vi "SetWavelength.vi"(8 "error in (no error)":errorcluster, 10 "Wavelength, nm":dbl=620.0, 11 "OPA in":refnum<class "OPA.lvclass">) -> (0 "error out":errorcluster, 3 "OPA out":refnum<class "OPA.lvclass">)   [LabVIEW 2017, in "OPA.lvclass"]
uses:
  OPA.lvclass
  Typedefs/PrivateEvents--OPA.SetWavelength.ctl
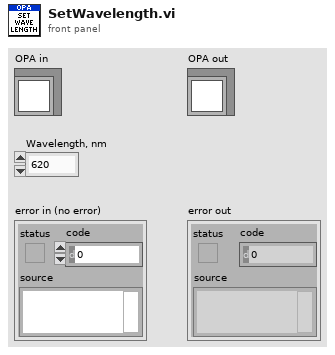
[diagram p1: front panel]
types:
  T1 = typedef "OPA.lvclass/PrivateEvents--OPA.SetWavelength.ctl" = cluster{"Wavelength, nm":dbl}
  T2 = typedef "OPA.lvclass/PrivateEvents--Cluster.ctl" = cluster{"SetWavelength":refnum<user-event>, "SetShutterState":refnum<user-event>}
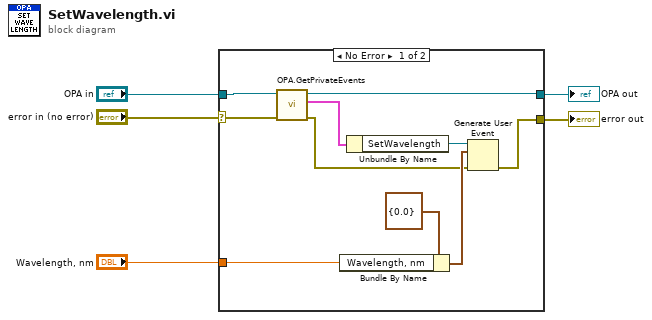
[diagram p0: block diagram]
diagram:
  n1 = case shown="No Error" "error in (no error)" {
    selector: "error in (no error)" -> [w9 w17]
    tunnel: [w7 w17] -> w4
    tunnel: [w6 w16] -> w2
    tunnel: "OPA in" -> [w15 w16]
    tunnel: "Wavelength, nm" -> [w10 _]
    frame No Error {
      n2 = call "OPA.GetPrivateEvents.vi"("error in (no error)"=w9, "OPA"=w15) -> ("error out"=w8:errorcluster, "Private Events"=w14:T2, "OPA out"=w6:refnum<class "OPA.lvclass">)  [unwired: 7 in]
      n3 = Bundle By Name(cluster=T1 {"Wavelength, nm"=0.0} ("SetWavelength"), "Wavelength, nm"=w10) -> (w12:T1)
      n4 = Unbundle By Name(w14) -> ("SetWavelength"=w13:refnum<user-event>)
      n5 = Generate User Event(user event=w13, event data cluster=w12, error in=w8) -> (error out=w7:errorcluster)  [unwired: 1 in, 1 out]
    }
    frame Error {
    }
  }
  "error out" <- w4
  "OPA out" <- w2
